vi "Callback Change Channel Name.vi"(6 "Variant":variant, 8 "error in (no error)":errorcluster, 9 "Old Values":string[][](array[string]), 10 "object ref in":T1, 11 "Table Change":T2) -> (0 "error out":errorcluster)   [LabVIEW 2014, in "Missing Plugin editor node.lvclass"]
doc: "This VI gets called automatically when changes are made to the 'Name' column of the table and must handle changes appropriately. Register this callback using the appropriate 'Define Column' VI from the Table API."
uses:
  Missing Plugin editor node.lvclass
  <vilib>/NI/DCAF/Tag Editor Core/Table API/Table Manager/Cell Change.ctl
  <vilib>/NI/DCAF/Tag Editor Core/Table API/Table Manager/object ref.ctl
  <vilib>/NI/DCAF/Tag Editor Core/Configuration Editor/Classes/Engine Parent/Engine Parent Editor Node.lvclass
  <vilib>/NI/DCAF/Tag Editor Core/Configuration Editor/Classes/Module editor node/module editor node.lvclass
  module/configuration/Missing Plugin configuration.lvclass
  module/configuration/Missing Plugin configuration.lvclass/Missing Plugin configuration.ctl
  <vilib>/NI/Tag Bus/tag/tag descriptor.lvclass/tag descriptor.ctl
  <vilib>/NI/Configuration Framework/serializable configuration/NISE_CEF_serializable configuration.lvclass/NISE_CEF_serializable configuration.ctl
  <vilib>/Utility/LVClass/Get LV Class Name.vi
  <vilib>/NI/Configuration Framework/error generator/NISE_error generator.vi
  module/configuration/Get Line Name.vi
  <vilib>/NI/Tag Bus Module Framework/module configuration/FindDuplicate.vi
  <vilib>/Utility/error.llb/Error Cluster From Error Code.vi
  <vilib>/NI/Tag Bus Module Framework/channel/TBM channel.lvclass
  <vilib>/NI/Module Execution Interface/Engine Configuration/engine configuration.lvclass
  <vilib>/NI/Tag Bus/tag/tag descriptor.lvclass
  <vilib>/NI/Configuration Framework/serializable configuration/NISE_CEF_serializable configuration.lvclass
  <vilib>/NI/DCAF/Tag Editor Core/Table API/Table Manager.lvlib
  <vilib>/NI/DCAF/Tag Editor Core/Table API/Table Manager/Table Manager.lvclass
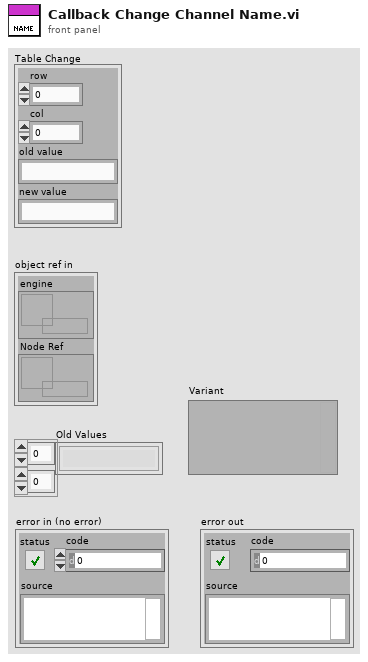
[diagram p1: front panel]
types:
  T1 = typedef "Table Manager.lvlib/Table Manager.lvclass/object ref.ctl" = cluster{"engine":refnum<data-value>, "Node Ref":refnum<data-value>}
  T2 = typedef "Table Manager.lvlib/Cell Change.ctl" = cluster{"row":i32, "col":i32, "old value":string, "new value":string}
  T3 = typedef "Missing Plugin configuration.lvclass/Line.ctl" = cluster{"channel":refnum<class "TBM channel.lvclass">}
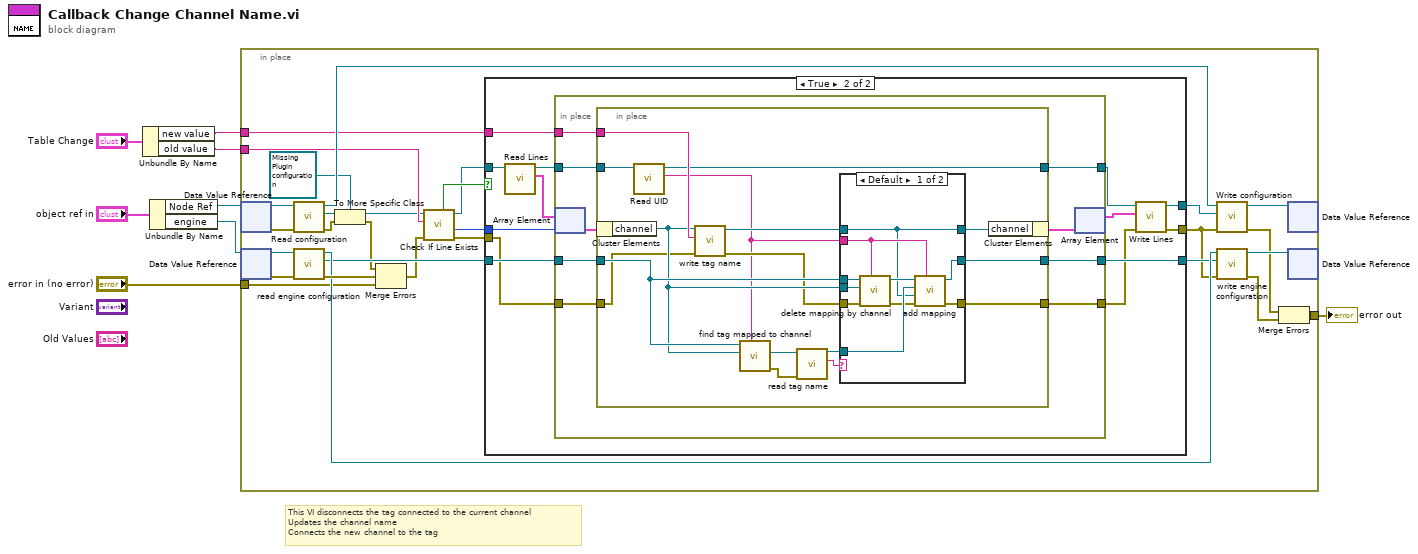
[diagram p0: block diagram]
diagram:
  # "This VI disconnects the tag connected to the current channel\nUpdates the channel name\nConnects the new channel to the tag"
  n1 = Unbundle By Name("Table Change") -> ("new value"=w1:string, "old value"=w2:string)
  n2 = Unbundle By Name("object ref in") -> ("Node Ref"=w5:refnum<data-value>, "engine"=w4:refnum<data-value>)
  n3 = in-place {
    in-place-border: [w29] -> w8
    in-place-border: "error in (no error)" -> [w25]
    in-place-border: w2 -> [w23]
    in-place-border: w1 -> [w20]
    n4 = in-place-dvr #1(w5) -> (w18:refnum<class "module editor node.lvclass">, w28:errorcluster)
    n5 = in-place-dvr #2(w4) -> (w36:refnum<class "Engine Parent Editor Node.lvclass">, w37:errorcluster)
    n6 = call-dynamic "Read configuration.vi"("error in"=w28, "NISE_CEF_serializable node in"=w18) -> ("error out"=w10:errorcluster, "configuration"=w26:refnum<class "NISE_CEF_serializable configuration.lvclass">, "NISE_CEF_serializable node out"=w27:refnum<class "module editor node.lvclass">)  [unwired: 7 in]
    n7 = call <vilib>:"read engine configuration.vi"("error in"=w37, "Engine Parent Editor Node in"=w36) -> ("error out"=w33:errorcluster, "engine configuration"=w15:refnum<class "engine configuration.lvclass">, "Engine Parent Editor Node out"=w32:refnum<class "Engine Parent Editor Node.lvclass">)  [unwired: 7 in]
    n8 = To More Specific Class(target class=refnum<class "Missing Plugin configuration.lvclass"> refnum ("tag bus configurable plugin module configuration"), reference=w26, error in=w10) -> (specific class reference=w17:refnum<class "Missing Plugin configuration.lvclass">, error out=w9:errorcluster)
    n9 = Merge Errors(w9, w33, w25) -> (w13:errorcluster)
    n10 = call-dynamic "Check If Line Exists.vi"("error in"=w13, "Name to Locate"=w23, "Missing Plugin configuration in"=w17) -> ("error out"=w14:errorcluster, "Index"=w21:i32, "Missing Plugin configuration out"=w12:refnum<class "Missing Plugin configuration.lvclass">, "Found?"=w19:bool)  [unwired: 4 in, 1 out]
    n11 = case shown="True" w19 {
      tunnel: [w40 w53] -> w22
      tunnel: w12 -> [w40 w52]
      tunnel: w21 -> [_ w49]
      tunnel: w20 -> [_ w48]
      tunnel: w15 -> [w39 w47]
      tunnel: [w39 w46] -> w16
      tunnel: [w38 w45] -> w11
      tunnel: w14 -> [w38 w43]
      frame False {
      }
      frame True {
        n12 = call "Read Lines.vi"("Missing Plugin configuration in"=w52) -> ("Lines"=w51:T3[], "Missing Plugin configuration out"=w42:refnum<class "Missing Plugin configuration.lvclass">)  [unwired: 8 in, 1 out]
        n13 = in-place {
          in-place-border: w48 -> [w60]
          in-place-border: w47 -> [w59]
          in-place-border: [w58] -> w46
          in-place-border: [w57] -> w44
          in-place-border: w43 -> [w56]
          in-place-border: w42 -> [w55]
          in-place-border: [w54] -> w41
          n14 = in-place-array #3(w51, w49) -> (w62:T3)
          n15 = in-place {
            in-place-border: w60 -> [w78]
            in-place-border: w59 -> [w76]
            in-place-border: [w77] -> w58
            in-place-border: [w68] -> w57
            in-place-border: w56 -> [w70]
            in-place-border: w55 -> [w66]
            in-place-border: [w65] -> w54
            n16 = in-place-cluster #4(w62) -> ("channel"=w75:refnum<class "TBM channel.lvclass">)
            n17 = call <vilib>:"Read UID.vi"("configuration in"=w66) -> ("instance id"=w67:string, "configuration out"=w65:refnum<class "Missing Plugin configuration.lvclass">)  [unwired: 8 in, 1 out]
            n18 = call <vilib>:"write tag name.vi"("error in"=w70, "name"=w78, "system tag in"=w75) -> ("error out"=w69:errorcluster, "system tag out"=w71:refnum<class "TBM channel.lvclass">)  [unwired: 7 in]
            n19 = call <vilib>:"find tag mapped to channel.vi"("owner"=w67, "channel"=w75, "engine configuration in"=w76) -> ("error out"=w63:errorcluster, "tag"=w74:refnum<class "tag descriptor.lvclass">)  [unwired: 6 in, 1 out]
            n20 = call <vilib>:"read tag name.vi"("error in"=w63, "system tag in"=w74) -> ("name"=w73:string, "system tag out"=w72:refnum<class "tag descriptor.lvclass">)  [unwired: 7 in, 1 out]
            n21 = case shown="Default" w73 {
              tunnel: [w87 w91] -> w77
              tunnel: w76 -> [w86 w91]
              tunnel: w67 -> [w85 _]
              tunnel: w75 -> [w84 _]
              tunnel: w72 -> [w83 _]
              tunnel: w71 -> [w79 w89]
              tunnel: [w81 w90] -> w68
              tunnel: w69 -> [w80 w90]
              tunnel: [w79 w89] -> w64
              frame Default {
                n22 = call <vilib>:"delete mapping by channel.vi"("owner ID"=w85, "error in"=w80, "channel"=w84, "engine configuration in"=w86) -> ("error out"=w82:errorcluster, "engine configuration out"=w88:refnum<class "engine configuration.lvclass">)  [unwired: 6 in]
                n23 = call-dynamic "add mapping.vi"("owner ID"=w85, "error in"=w82, "channel"=w79, "tag descriptor"=w83, "engine configuration"=w88) -> ("error out"=w81:errorcluster, "engine configuration out"=w87:refnum<class "engine configuration.lvclass">)  [unwired: 5 in]
              }
              frame "" {
              }
            }
            n24 = in-place-cluster #4("channel"=w64) -> (w61:T3)
          }
          n25 = in-place-array #3(w61) -> (w50:T3[])  [unwired: 1 out]
        }
        n26 = call "Write Lines.vi"("error in (no error)"=w44, "Lines"=w50, "Missing Plugin configuration in"=w41) -> ("error out"=w45:errorcluster, "Missing Plugin configuration out"=w53:refnum<class "Missing Plugin configuration.lvclass">)  [unwired: 7 in]
      }
    }
    n27 = call-dynamic "Write configuration.vi"("error in"=w11, "configuration"=w22, "NISE_CEF_serializable node in"=w27) -> ("error out"=w30:errorcluster, "NISE_CEF_serializable node out"=w34:refnum<class "module editor node.lvclass">)  [unwired: 7 in]
    n28 = call <vilib>:"write engine configuration.vi"("error in"=w11, "engine configuration"=w16, "Engine Parent Editor Node in"=w32) -> ("error out"=w31:errorcluster, "Engine Parent Editor Node out"=w35:refnum<class "Engine Parent Editor Node.lvclass">)  [unwired: 7 in]
    n29 = Merge Errors(w30, w31) -> (w29:errorcluster)
    n30 = in-place-dvr #1(w34) -> ()  [unwired: 2 out]
    n31 = in-place-dvr #2(w35) -> ()  [unwired: 2 out]
  }
  "error out" <- w8
